vi "LMS_Calibrate.vi"(6 "bw":dbl, 7 "flags":u16, 8 "error in (no error)":errorcluster, 9 "chan":u64, 10 "dir_tx":u8, 11 "device_In":i64) -> (0 "error out":errorcluster, 3 "device_Out":i64)   [LabVIEW 2013, in "LMS_LV_Drv.lvlib"]
uses:
  LMS_LV_Drv.lvlib
  Program Files/PothosSDR/bin/LimeSuite.dll
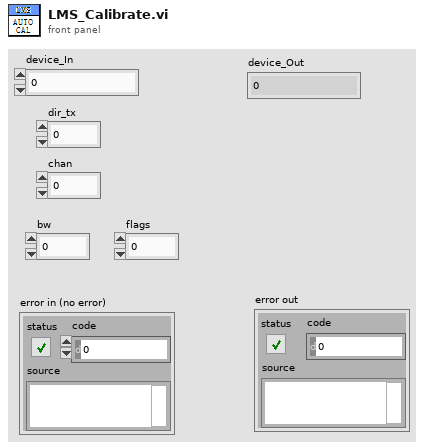
[diagram p1: front panel]
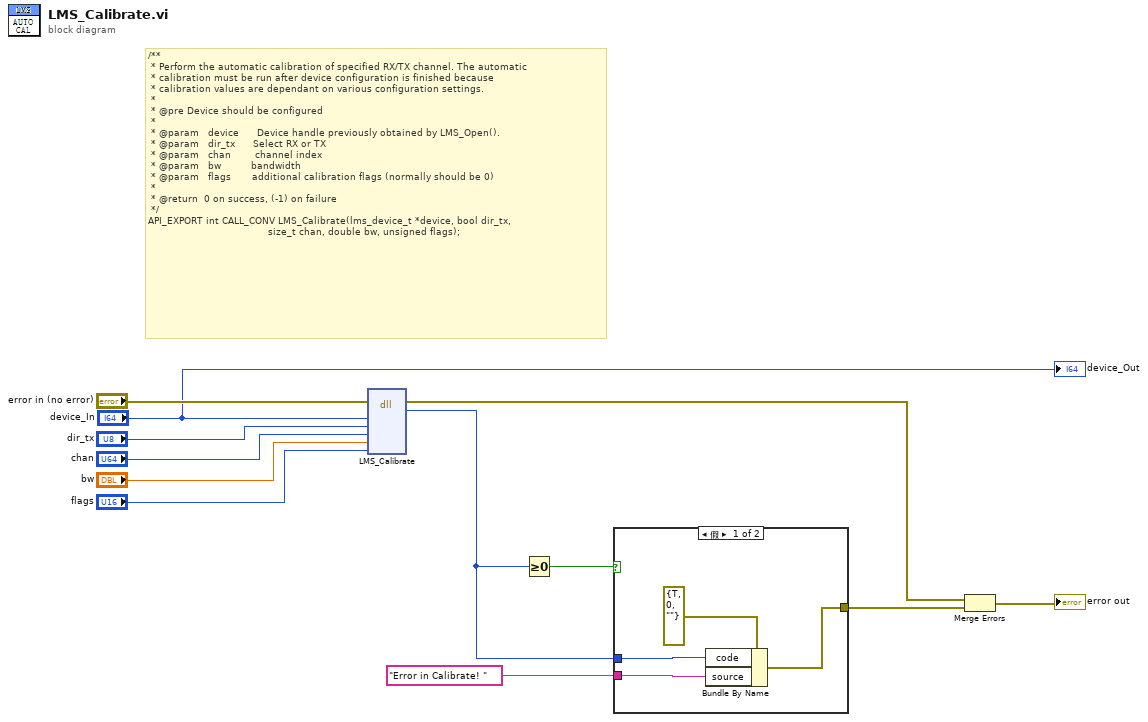
[diagram p0: block diagram]
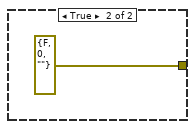
[diagram p2: hidden frame]
diagram:
  # "/**\n * Perform the automatic calibration of specified RX/TX channel. The automatic\n * calibration must be run after device configuration is finished because\n * calibration values are dependant on various configuration settings.\n *\n * @pre Device should be configured\n *\n * @param   device      Device handle previously obtained by LMS_Open().\n * @param   dir_tx      Select RX or TX\n * @param   chan        channel index\n * @param   bw          bandwidth\n * @param   flags       additional calibration flags (normally should be 0)\n *\n * @return  0 on success, (-1) on failure\n */\nAPI_EXPORT int CALL_CONV LMS_Calibrate(lms_device_t *device, bool dir_tx,\n                                        size_t chan, double bw, unsigned flags);"
  n1 = dll-call lib="C:/Program Files/PothosSDR/bin/LimeSuite.dll" fn="LMS_Calibrate"(error in="error in (no error)", "device"="device_In", "dir_tx"="dir_tx", "chan"="chan", "bw"="bw", "flags"="flags") -> (error out=w2:errorcluster, "return type"=w3:i32)  [unwired: 7 in, 1 out]
  n2 = Greater Or Equal To 0?(x=w3) -> (x >= 0?=w6:bool)
  n3 = case shown="假" w6 {
    tunnel: [w15 errorcluster {"status"=FALSE, "code"=0, "source"=""} ("error in")] -> w4
    tunnel: w3 -> [w14 _]
    tunnel: "Error in Calibrate! " ("source") -> [w13 _]
    frame False {
      n4 = Bundle By Name(cluster=errorcluster {"status"=TRUE, "code"=0, "source"=""} ("error in"), "code"=w14, "source"=w13) -> (w15:errorcluster)
    }
    frame True {
    }
  }
  n5 = Merge Errors(w2, w4) -> (→"error out":errorcluster)
  "device_Out" <- "device_In"
